vi "Read Status.vi"(6 "bytes to read":i32=4, 8 "error in (no error)":errorcluster, 9 "Status offset":u64, 10 "Read config instead":bool, 11 "RP Instrument in":refnum<class "RP Instrument.lvclass">) -> (0 "error out":errorcluster, 2 "Status response":u32=1 format="0x%x (%d)", 3 "RP Instrument out":refnum<class "RP Instrument.lvclass">)   [LabVIEW 2024, in "RP Instrument.lvclass"]
uses:
  RP Instrument.lvclass
  RP Instrument.lvclass/RP Instrument.ctl
  RP Communicator/RP Communicator.lvclass
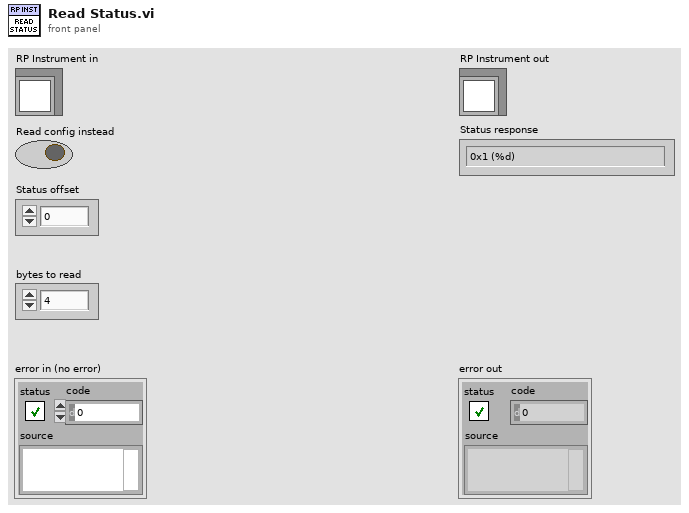
[diagram p1: front panel]
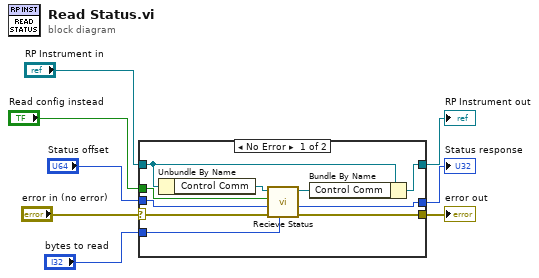
[diagram p0: block diagram]
diagram:
  n1 = case shown="No Error" "error in (no error)" {
    selector: "error in (no error)" -> [w16 w20]
    tunnel: [w15 w20] -> w7
    tunnel: [w14 w19] -> w5
    tunnel: "RP Instrument in" -> [w18 w19]
    tunnel: "Status offset" -> [w12 _]
    tunnel: "Read config instead" -> [w11 _]
    tunnel: "bytes to read" -> [w10 _]
    tunnel: [w9 _] -> w1
    frame No Error {
      n2 = Unbundle By Name(w18) -> ("Control Comm"=w17:refnum<class "RP Communicator.lvclass">)
      n3 = call-dynamic "Recieve Status.vi"("bytes to read"=w10, "error in (no error)"=w16, "Status offset"=w12, "Read config instead"=w11, "RP Communicator in"=w17) -> ("error out"=w15:errorcluster, "Status response"=w9:u32, "RP Communicator out"=w13:refnum<class "RP Communicator.lvclass">)  [unwired: 4 in]
      n4 = Bundle By Name(cluster=w18, "Control Comm"=w13) -> (w14:refnum<class "RP Instrument.lvclass">)
    }
    frame Error {
    }
  }
  "error out" <- w7
  "RP Instrument out" <- w5
  "Status response" <- w1
